vi "GetHeadFromPurgeSwitchName.vi"(11 "input string":string="Purge Switch - R2") -> (2 "whole match":string, 3 "output 1":T1=enum."1")   [LabVIEW 2022 SP3]
uses:
  Typedefs/PrinterHeads--Enum.ctl
  <vilib>/regexp/Match Regular Expression.xnode
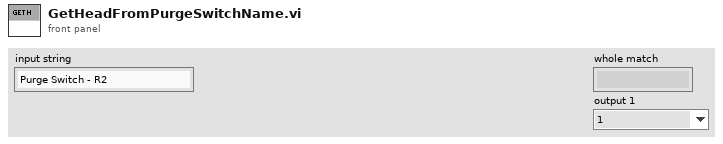
[diagram p1: front panel]
types:
  T1 = typedef "PrinterHeads--Enum.ctl" = enum16{"-1", "1", "2", "3", "4", "5", "6"}
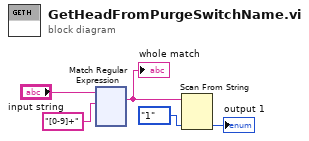
[diagram p0: block diagram]
diagram:
  n1 = xnode "Match Regular Expression"("input string"="input string", "regular expression"="[0-9]+") -> ("whole match"=w2:string)  [unwired: 4 in, 4 out]
  "whole match" <- w2
  n2 = Scan From String(input string=w2, default 1=PrinterHeads--Enum."1" ("Head")) -> (output 1=→"output 1":T1)  [unwired: 3 in, 3 out]
